vi "pcupdate.vi"() -> ()   [LabVIEW 2013]
uses:
  <vilib>/httpClient/LabVIEWHTTPClient.lvlib
  <vilib>/zip/NI_Unzip.lvlib
panel:
  out "Nahrani neceho probehlo":bool
  out "error out":errorcluster
  out "Unzipped files":path[](array[path])
  in  "url":string
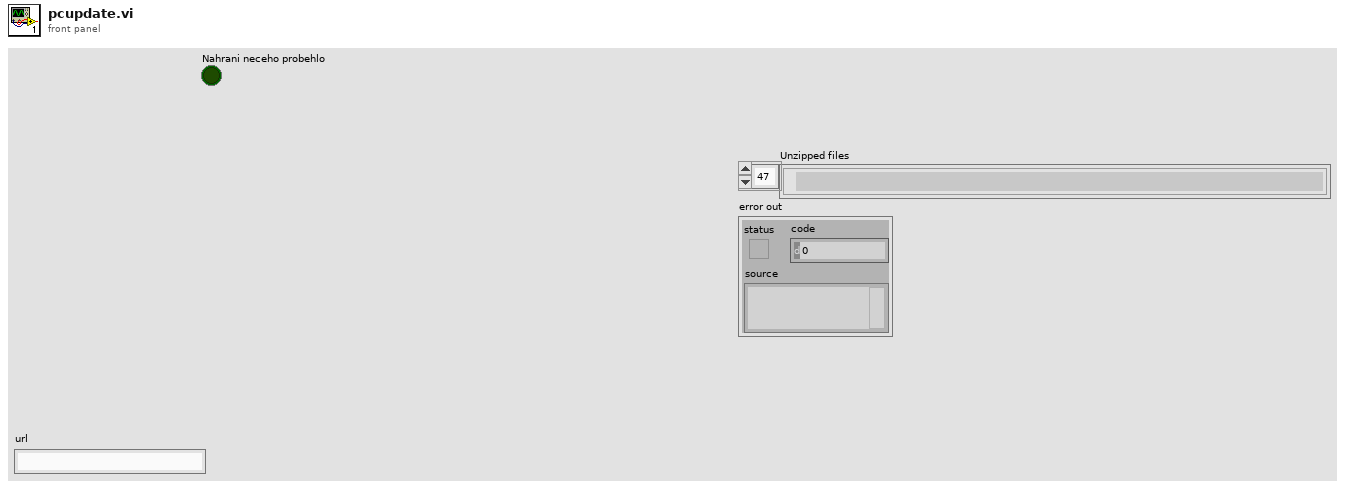
[diagram p1: front panel]
types:
  T1 = typedef "LVHSConnector.ctl" = refnum<class "BrickReference.lvclass">
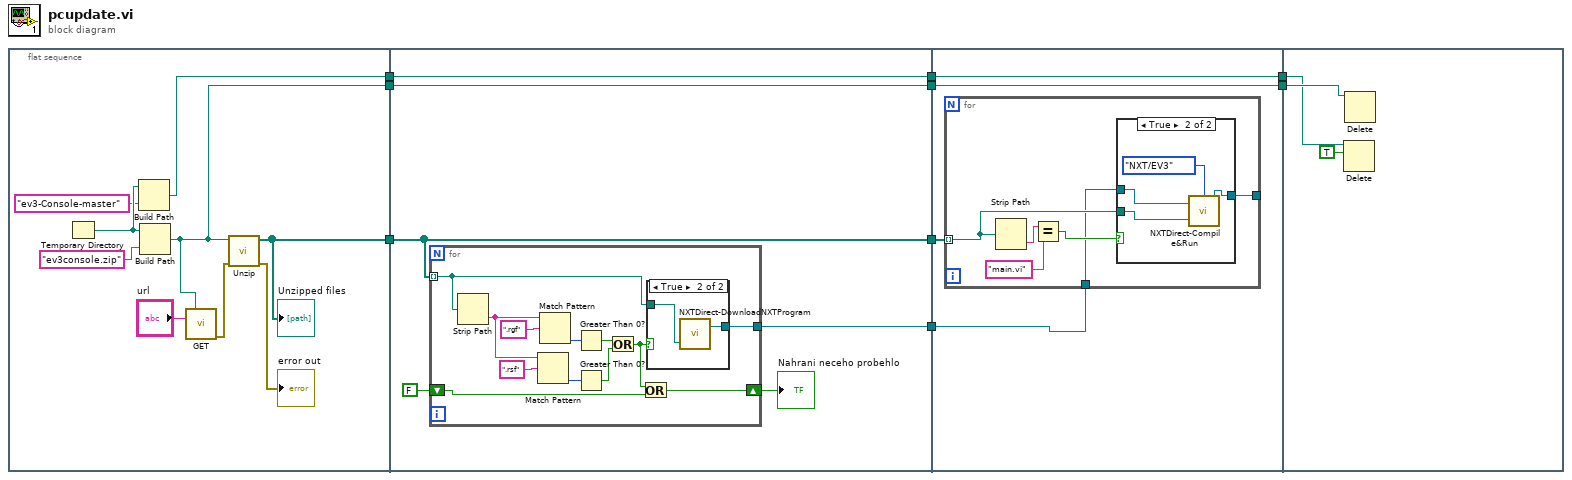
[diagram p0: block diagram]
diagram:
  n1 = flat-sequence {
    tunnel: [w14] -> w9
    tunnel: [w13] -> w6
    tunnel: [w10] -> w1
    tunnel: w9 -> [w21]
    tunnel: [w24] -> w8
    tunnel: [w21] -> w7
    tunnel: w6 -> [w20]
    tunnel: [w20] -> w5
    tunnel: [w19] -> w2
    tunnel: w1 -> [w19]
    tunnel: w8 -> [w41]
    tunnel: w7 -> [w42]
    tunnel: w5 -> [w40]
    tunnel: [w40] -> w4
    tunnel: [w39] -> w3
    tunnel: w2 -> [w39]
    tunnel: w4 -> [w56]
    tunnel: w3 -> [w55]
    frame #0 {
      n2 = Temporary Directory() -> (w12:path)
      n3 = Build Path(base path=w12, name or relative path="ev3-Console-master") -> (appended path=w10:path)
      n4 = Build Path(base path=w12, name or relative path="ev3console.zip") -> (appended path=w13:path)
      n5 = call <vilib>:"GET.vi"("output file"=w13, "url"="url") -> ("error out"=w17:errorcluster)  [unwired: 10 in, 3 out]
      n6 = call <vilib>:"Unzip.vi"("error in (no error)"=w17, "Zip file"=w13) -> ("error out"=→"error out":errorcluster, "Unzipped files"=w14:path[])  [unwired: 7 in, 1 out]
      "Unzipped files" <- w14
    }
    frame #1 {
      n7 = for {
        tunnel: w21 -> [w35] mode=indexing
        tunnel: [w36] -> w24
        shift-right: [w27] -> w22
        shift-left: FALSE -> [w26]
        n8 = Strip Path(path=w35) -> (name=w30:string)  [unwired: 1 out]
        n9 = Match Pattern(string=w30, regular expression=".rsf") -> (offset past match=w32:i32)  [unwired: 1 in, 3 out]
        n10 = Match Pattern(string=w30, regular expression=".rgf") -> (offset past match=w34:i32)  [unwired: 1 in, 3 out]
        n11 = Greater Than 0?(x=w34) -> (x > 0?=w33:bool)
        n12 = Greater Than 0?(x=w32) -> (x > 0?=w31:bool)
        n13 = Or(x=w33, y=w31) -> (x .or. y?=w25:bool)
        n14 = Or(x=w25, y=w26) -> (x .or. y?=w27:bool)
        n15 = case shown="True" w25 {
          tunnel: [_ w38] -> w36
          tunnel: w35 -> [_ w37]
          frame False {
          }
          frame True {
            n16 = call <vilib>:"NXTDirect-DownloadNXTProgram.vi"("File Path"=w37) -> ("NXT/EV3"=w38:T1)  [unwired: 2 in, 1 out]
          }
        }
      }
      "Nahrani neceho probehlo" <- w22
    }
    frame #2 {
      n17 = for {
        tunnel: w42 -> [w46] mode=indexing
        tunnel: [w48] -> _
        tunnel: w41 -> [w43]
        n18 = Strip Path(path=w46) -> (name=w45:string)  [unwired: 1 out]
        n19 = Equal?(x=w45, y="main.vi" ("regular expression")) -> (x = y?=w44:bool)
        n20 = case shown="True" w44 {
          tunnel: [w49 w52] -> w48
          tunnel: w46 -> [_ w53]
          tunnel: w43 -> [w49 w51]
          frame False {
          }
          frame True {
            n21 = call <vilib>:"NXTDirect-Compile&Run.vi"("VI Path"=w53, "NXT/EV3"=w51, "Target"=enum16{"NXT/EV3", "PC"}."NXT/EV3") -> ("NXT/EV3"=w52:T1)  [unwired: 2 in]
          }
        }
      }
    }
    frame #3 {
      n22 = Delete(path (use dialog)=w55, entire hierarchy (F)=TRUE) -> ()  [unwired: 3 in, 3 out]
      n23 = Delete(path (use dialog)=w56) -> ()  [unwired: 4 in, 3 out]
    }
  }
